vi "New_camera_connection_testcode.vi"(8 "error in":errorcluster, 10 "CAM_ID2":i32, 11 "CAM_ID1":i32) -> (0 "CAM2 Model":enum16{"a2A5328-15ucBAS", "acA1920-155uc"}(ring), 1 "CAM1 Model":enum16{"a2A5328-15ucBAS", "acA1920-155uc"}(ring), 2 "CAM2":string, 3 "CAM1":string, 4 "error out":errorcluster)   [LabVIEW 2024]
uses:
  <vilib>/vision/driver/NI_Vision_Acquisition_Software.lvlib
panel:
  out "Array 3":bool[](array[boolean])
  out "Array 2":string[](array[string])
  out "Array":u32[](array[numeric])
  out "ModelNameCAM1":string
  out "ModelNameCAM2":string
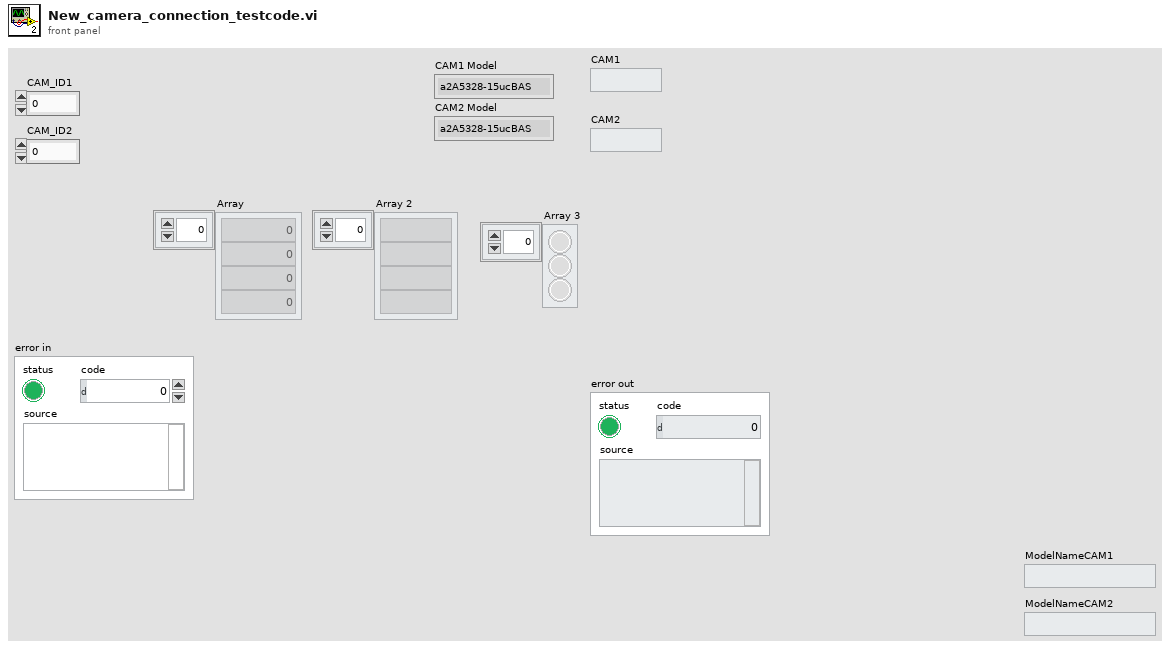
[diagram p1: front panel]
types:
  T1 = cluster{"Type":u32, "Version":u32, "Flags":u32, "SerialNumberHigh":u32, "SerialNumberLow":u32, "BusType":u32, "InterfaceName":string, "VendorName":string, "ModelName":string, "CameraFileName":string, "CameraAttributeURL":string}[]
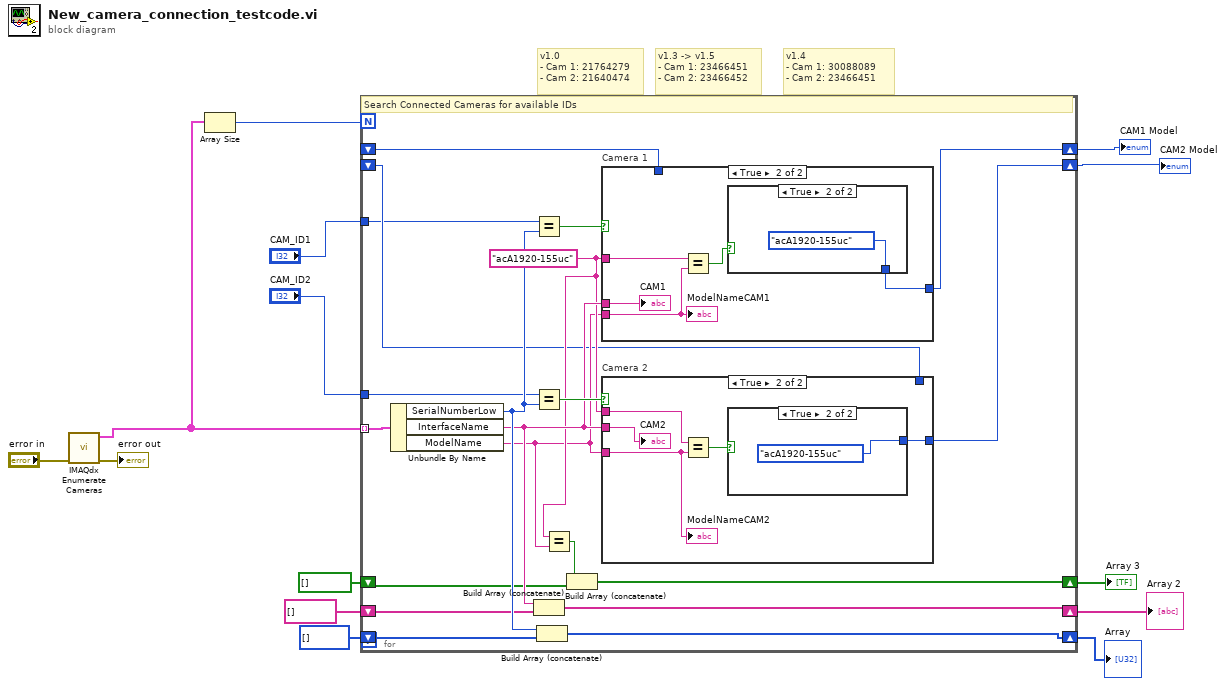
[diagram p0: block diagram]
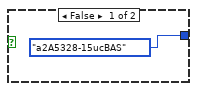
[diagram p3: hidden frame]
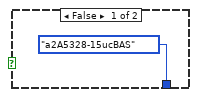
[diagram p5: hidden frame]
diagram:
  # "v1.4\n- Cam 1: 30088089 \n- Cam 2: 23466451"
  # "v1.3 -> v1.5\n- Cam 1: 23466451 \n- Cam 2: 23466452"
  # "v1.0\n- Cam 1: 21764279 \n- Cam 2: 21640474"
  n1 = call <vilib>:"IMAQdx Enumerate Cameras.vi"("error in"="error in") -> ("error out"=→"error out":errorcluster, "Camera Information Array"=w13:T1)  [unwired: 9 in]
  n2 = Array Size(array=w13) -> (size(s)=w14:i32)
  n3 = for {
    N: w14 -> [_]
    tunnel: w13 -> [w34] mode=indexing
    tunnel: "CAM_ID1" -> [w16]
    tunnel: "CAM_ID2" -> [w15]
    shift-right: [w29] -> w10
    shift-left: u32[] [] -> [w30]
    shift-right: [w28] -> w8
    shift-left: string[] [] -> [w27]
    shift-right: [w22] -> w5
    shift-left: bool[] [] -> [w21]
    shift-right: [w19] -> w3
    shift-left: _ -> [w17]
    shift-right: [w20] -> w4
    shift-left: _ -> [w18]
    w25 = "acA1920-155uc"
    # "Search Connected Cameras for available IDs"
    n4 = Unbundle By Name(w34) -> ("SerialNumberLow"=w31:u32, "InterfaceName"=w26:string, "ModelName"=w24:string)
    n5 = Equal?(x=w16, y=w31) -> (x = y?=w33:bool)
    n6 = Equal?(x=w15, y=w31) -> (x = y?=w32:bool)
    n7 = Build Array (concatenate)(w26, w27) -> (w28:string[])
    n8 = Build Array (concatenate)(w31, w30) -> (w29:u32[])
    n9 = Equal?(x=w25, y=w24) -> (x = y?=w23:bool)
    n10 = Build Array (concatenate)(w23, w21) -> (w22:bool[])
    n11 = case "Camera 1" shown="True" w33 {
      tunnel: w26 -> [_ w48]
      tunnel: w24 -> [_ w47]
      tunnel: w25 -> [_ w46]
      tunnel: [w43 w44] -> w20
      tunnel: w18 -> [w43 _]
      frame False {
      }
      frame True {
        n12 = Equal?(x=w46, y=w47) -> (x = y?=w45:bool)
        n13 = case shown="True" w45 {
          tunnel: [enum16{"a2A5328-15ucBAS", "acA1920-155uc"}."a2A5328-15ucBAS" ("CAM1 Model") enum16{"a2A5328-15ucBAS", "acA1920-155uc"}."acA1920-155uc" ("CAM1 Model")] -> w44
          frame False {
          }
          frame True {
          }
        }
        "CAM1" <- w48
        "ModelNameCAM1" <- w47
      }
    }
    n14 = case "Camera 2" shown="True" w32 {
      tunnel: w26 -> [_ w40]
      tunnel: w24 -> [_ w39]
      tunnel: w25 -> [_ w38]
      tunnel: [w35 w36] -> w19
      tunnel: w17 -> [w35 _]
      frame False {
      }
      frame True {
        n15 = Equal?(x=w38, y=w39) -> (x = y?=w37:bool)
        n16 = case shown="True" w37 {
          tunnel: [enum16{"a2A5328-15ucBAS", "acA1920-155uc"}."a2A5328-15ucBAS" ("CAM2 Model") enum16{"a2A5328-15ucBAS", "acA1920-155uc"}."acA1920-155uc" ("CAM2 Model")] -> w36
          frame False {
          }
          frame True {
          }
        }
        "CAM2" <- w40
        "ModelNameCAM2" <- w39
      }
    }
  }
  "Array" <- w10
  "Array 2" <- w8
  "Array 3" <- w5
  "CAM1 Model" <- w4
  "CAM2 Model" <- w3
